vi "Load-sequences-with-dialog.vi"(8 "error in (no error)":errorcluster, 11 "Object ref in":T1) -> (0 "error out":errorcluster, 3 "Object ref out":T1)   [LabVIEW 2013, in "PowderDeposition.lvlib" / "PD-Main.lvclass"]
uses:
  PD-Main.lvclass
  Object-reference.ctl
  PD-Main.lvclass/PD-Main.ctl
  Client-status.ctl
  Custom-errors.ctl
  Assembly/Motor-assembly.lvclass
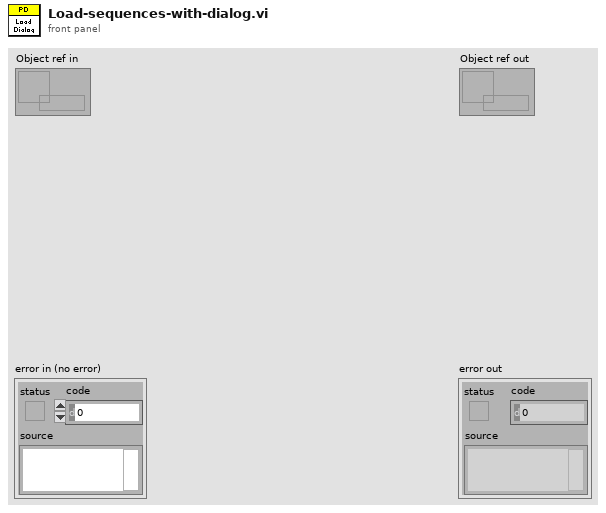
[diagram p1: front panel]
types:
  T1 = typedef "PowderDeposition.lvlib/PD-Main.lvclass/Object-reference.ctl" = refnum<data-value>
  T2 = typedef "PowderDeposition.lvlib/PD-Main.lvclass/Client-status.ctl" = enum16{"Idle", "Initialized", "Configured", "Activated", "Started", "Paused", "Stopped", "Reset", "Error", "Exited"}
  T3 = typedef "PowderDeposition.lvlib/PD-Main.lvclass/Custom-errors.ctl" = enum16{"Not implemented", "Command not recognized", "Invalid input", "Timeout", "Load file failed", "Action failed", "Action invalid", "Motor inactive", "Not in range", "Unsafe state"}
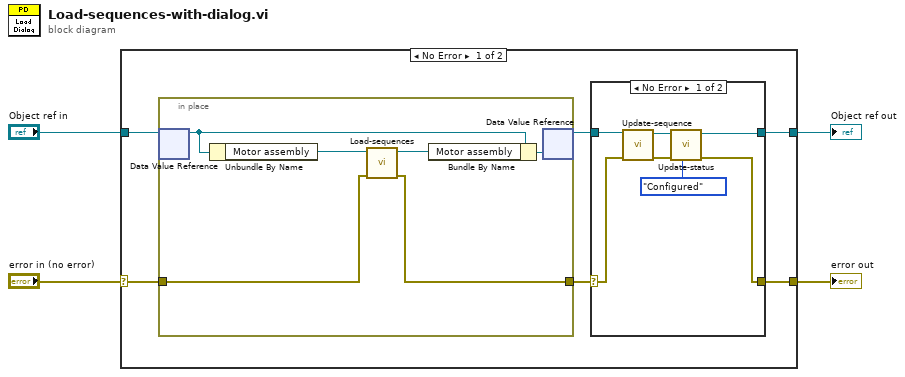
[diagram p0: block diagram]
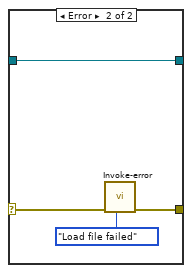
[diagram p2: hidden frame]
diagram:
  n1 = case shown="No Error" "error in (no error)" {
    selector: "error in (no error)" -> [w9 w29]
    tunnel: [w5 w29] -> w3
    tunnel: [w7 w28] -> w1
    tunnel: "Object ref in" -> [w10 w28]
    frame No Error {
      n2 = in-place {
        in-place-border: w9 -> [w27]
        in-place-border: [w22] -> w6
        n3 = in-place-dvr #1(w10) -> (w25:refnum<class "PD-Main.lvclass">)  [unwired: 1 out]
        n4 = Unbundle By Name(w25) -> ("Motor assembly"=w26:refnum<class "Motor-assembly.lvclass">)
        n5 = call "Load-sequences.vi"("error in (no error)"=w27, "Available motors in"=w26) -> ("error out"=w22:errorcluster, "Available motors out"=w23:refnum<class "Motor-assembly.lvclass">)  [unwired: 8 in]
        n6 = Bundle By Name(cluster=w25, "Motor assembly"=w23) -> (w24:refnum<class "PD-Main.lvclass">)
        n7 = in-place-dvr #1(w24) -> (w8:T1)  [unwired: 1 out]
      }
      n8 = case shown="No Error" w6 {
        selector: w6 -> [w11 w19]
        tunnel: w8 -> [w14 w18]
        tunnel: [w16 w21] -> w5
        tunnel: [w17 w18] -> w7
        frame No Error {
          n9 = call "Update-sequence.vi"("error in (no error)"=w11, "Object ref in"=w14) -> ("error out"=w12:errorcluster, "Object ref out"=w13:T1)  [unwired: 8 in]
          n10 = call "Update-status.vi"("Status"=Client-status."Configured", "error in (no error)"=w12, "Object ref in"=w13) -> ("error out"=w16:errorcluster, "Object ref out"=w17:T1)  [unwired: 7 in]
        }
        frame Error {
          n11 = call "Invoke-error.vi"("Error"=Custom-errors."Load file failed", "error in (no error)"=w19) -> ("error out"=w21:errorcluster)  [unwired: 9 in]
        }
      }
    }
    frame Error {
    }
  }
  "error out" <- w3
  "Object ref out" <- w1
